vi "Overlay.vi"(8 "error in (no error)":errorcluster, 10 "Image In":T1, 11 "Overlay Base in":refnum<class "Analyze Results Energy.lvclass">) -> (0 "error out":errorcluster, 2 "Image out":T1, 3 "Overlay Base out":refnum<class "Analyze Results Energy.lvclass">)   [LabVIEW 2020, in "Analyze Results Energy.lvclass"]
uses:
  Analyze Results Energy.lvclass
  C:/POLARIS Programme/POLARIS-AS-3-Cams/Submodules/HIJ Vision/Analyze/Results and Overlays/Results Base/Analyze Results Base.lvclass
  <vilib>/vision/Image Controls.llb/IMAQ Image.ctl
  Analyze Results Energy.lvclass/Analyze Results Energy.ctl
  Results Base/Analyze Results Base.lvclass/Analyze Results Base.ctl
  Read Energy.vi
  Results Base/Read Font, Size & Style.vi
  Results Base/Read Position.vi
  Results Base/Read Overlay colors.vi
  Results Base/Read Overlay_.vi
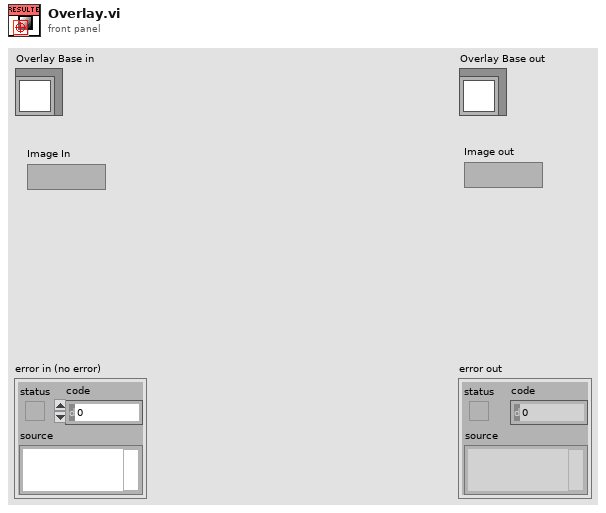
[diagram p1: front panel]
types:
  T1 = typedef "IMAQ Image.ctl" = refnum<image>
  T2 = cluster{"Desired Font (Application)":enum16{"User-specified Font", "Application Font", "System Font", "Dialog Font"}, "[User-specified Font]":cluster{"Font Name":string, "Size":i16, "Strikeout?":bool, "Italic?":bool, "Underline?":bool, "Outline?":bool, "Shadow?":bool, "Bold?":bool, "Rotation Angle":dbl}, "Horizontal Alignment":i16, "Vertical Alignment":i16}
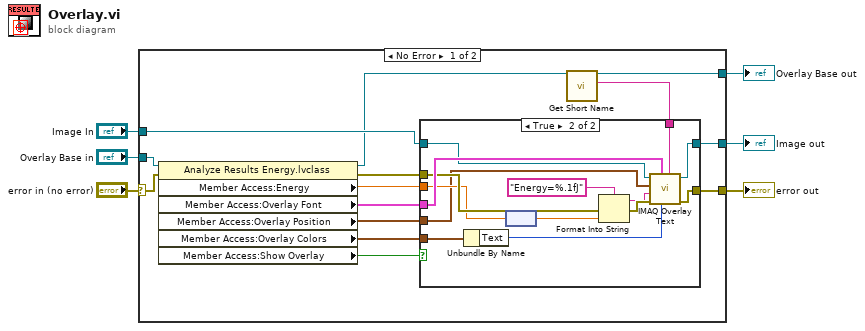
[diagram p0: block diagram]
diagram:
  n1 = case shown="No Error" "error in (no error)" {
    selector: "error in (no error)" -> [w10 w39]
    tunnel: "Overlay Base in" -> [w9 w38]
    tunnel: "Image In" -> [w20 w37]
    tunnel: [w8 w38] -> w3
    tunnel: [w17 w37] -> w2
    tunnel: [w14 w39] -> w1
    frame No Error {
      n2 = property class="Analyze Results Energy.lvclass"(reference=w9, error in=w10) -> (reference out=w18:refnum<class "Analyze Results Energy.lvclass">, error out=w19:errorcluster, "Member Access:Energy"=w16:dbl[unit], "Member Access:Overlay Font"=w11:T2, "Member Access:Overlay Position"=w15:cluster{"x":i16, "y":i16}, "Member Access:Overlay Colors"=w13:cluster{"Border":u32, "Text":u32}, "Member Access:Show Overlay"=w12:bool)
      n3 = call-dynamic "Get Short Name.vi"("Analyze Results Base in"=w18) -> ("Short Name"=w7:string, "Analyze Results Base out"=w8:refnum<class "Analyze Results Energy.lvclass">)  [unwired: 8 in, 1 out]
      n4 = case shown="True" w12 {
        tunnel: w20 -> [w22 w29]
        tunnel: [w22 w32] -> w17
        tunnel: w19 -> [w21 w28]
        tunnel: [w21 w31] -> w14
        tunnel: w11 -> [_ w34]
        tunnel: w16 -> [_ w27]
        tunnel: w15 -> [_ w26]
        tunnel: w13 -> [_ w25]
        tunnel: w7 -> [_ w23]
        frame False {
        }
        frame True {
          n5 = Unbundle By Name(w25) -> ("Text"=w30:u32)
          n6 = node(w27) -> (w24:dbl)
          n7 = Format Into String(format string="Energy=%.1fJ", error in=w28, w24) -> (resulting string=w33:string, error out=w35:errorcluster)  [unwired: 1 in]
          n8 = call "IMAQ Overlay Text"("Group"=w23, "Text Color (black)"=w30, "Font, Size & Style"=w34, "error in (no error)"=w35, "String"=w33, "Origin"=w26, "Image"=w29) -> ("error out"=w31:errorcluster, "Image Out"=w32:T1)  [unwired: 3 in]
        }
      }
    }
    frame Error {
    }
  }
  "error out" <- w1
  "Overlay Base out" <- w3
  "Image out" <- w2
